vi "CHROMA Set Phase Shift.vi"(8 "Error In":errorcluster, 9 "Value":i32=180, 10 "Phase Shift Lines":T1, 11 "CHROMA VISA In":refnum<visa-resource-name>) -> (0 "Error Out":errorcluster, 3 "CHROMA VISA Out":refnum<visa-resource-name>)   [LabVIEW 2018]
uses:
  Type Definition/CHROMA Phase Shift Lines.ctl
  Type Definition/CHROMA Build CMD Type.ctl
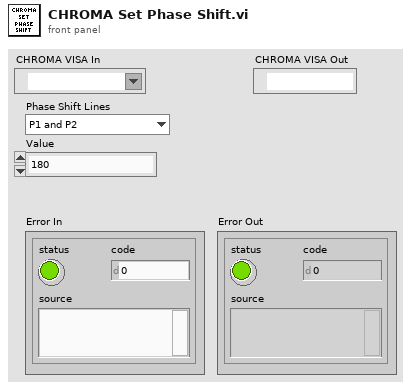
[diagram p1: front panel]
types:
  T1 = typedef "CHROMA Phase Shift Lines.ctl" = enum16{"P1 and P2", "P1 and P3"}
  T2 = typedef "CHROMA Build CMD Type.ctl" = enum16{"Value DBL", "Value I32", "String"}
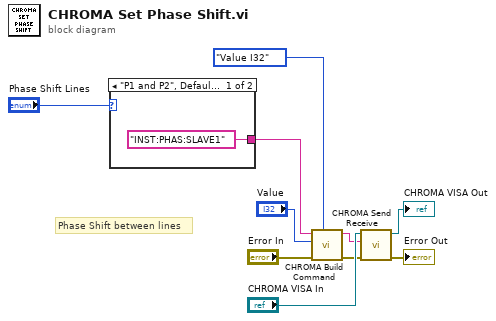
[diagram p0: block diagram]
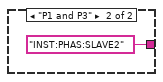
[diagram p2: hidden frame]
diagram:
  # "Phase Shift between lines"
  n1 = case shown="\"P1 and P2\", Default" "Phase Shift Lines" {
    tunnel: ["INST:PHAS:SLAVE1" ("string to write") "INST:PHAS:SLAVE2" ("string to write")] -> w9
    frame "P1 and P2", Default {
    }
    frame "P1 and P3" {
    }
  }
  n2 = call "CHROMA Build Command.vi"("Build Type"=CHROMA_Build_CMD_Type."Value I32", "Error In"="Error In", "Value"="Value", "Partial Command"=w9) -> ("Error Out"=w4:errorcluster, "Chroma Command"=w5:string)  [unwired: 6 in]
  n3 = call "CHROMA Send Receive.vi"("error in (no error)"=w4, "Send Command"=w5, "CHROMA VISA In"="CHROMA VISA In") -> ("error out"=→"Error Out":errorcluster, "CHROMA VISA Out"=→"CHROMA VISA Out":refnum<visa-resource-name>)  [unwired: 6 in, 1 out]
